vi "Delete.vi"(8 "error in":errorcluster caption="错误输入（无错误）", 10 "Data":variant, 11 "PanelRootNode 输入":refnum<class "PanelRootNode.lvclass"> caption="DNL_LabVIEW Object in") -> (0 "error out":errorcluster caption="错误输出", 3 "PanelRootNode 输出":refnum<class "PanelRootNode.lvclass"> caption="DNL_LabVIEW Object out")   [LabVIEW 2013, in "PanelRootNode.lvclass"]
uses:
  PanelRootNode.lvclass
  PanelObject/PanelObject.lvclass
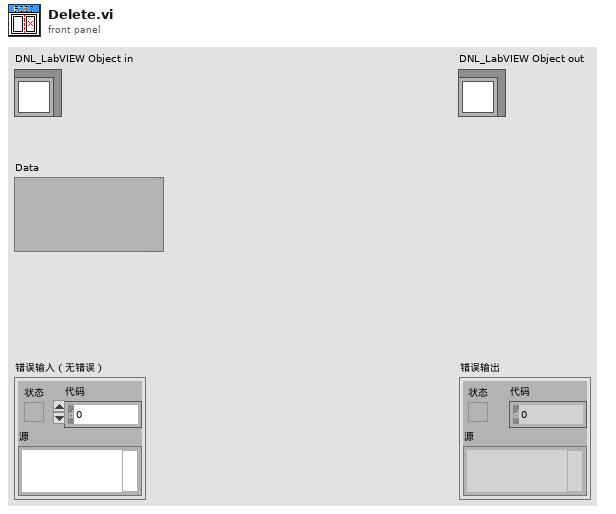
[diagram p1: front panel]
types:
  T1 = cluster{"Node*":refnum<data-value>, "AbortVI":bool}
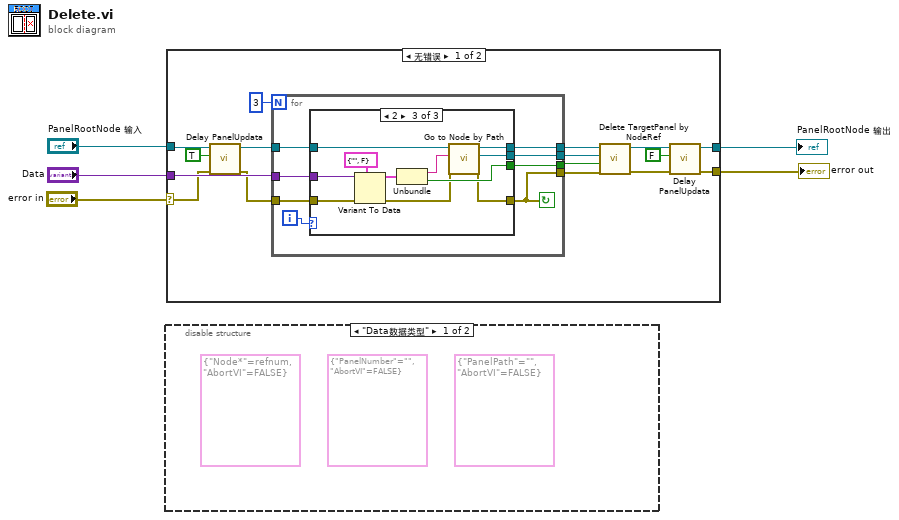
[diagram p0: block diagram]
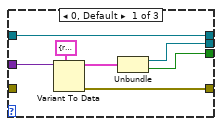
[diagram p3: hidden frame]
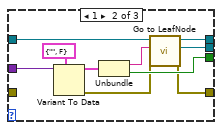
[diagram p4: hidden frame]
diagram:
  n1 = disable-structure shown="\"Data数据类型\"" {
    frame condition #0 {
      (unwired) cluster{"PanelPath":string, "AbortVI":bool} {"PanelPath"="", "AbortVI"=FALSE}
      (unwired) cluster{"PanelNumber":string, "AbortVI":bool} {"PanelNumber"="", "AbortVI"=FALSE}
      (unwired) T1 {"Node*"=refnum, "AbortVI"=FALSE}
    }
    frame condition #1 (active) {
    }
  }
  n2 = case shown="无错误" "error in" {
    selector: "error in" -> [w13 w59]
    tunnel: [w8 w59] -> w4
    tunnel: [w7 w58] -> w2
    tunnel: "PanelRootNode 输入" -> [w15 w58]
    tunnel: "Data" -> [w20 _]
    frame No Error {
      n3 = call "Delay PanelUpdata.vi"("error in (no error)"=w13, "延迟前面板更新"=TRUE, "PanelRootNode 输入"=w15) -> ("error out"=w12:errorcluster, "PanelRootNode 输出"=w14:refnum<class "PanelRootNode.lvclass">)  [unwired: 7 in]
      n4 = for {
        N: 3 -> [_]
        tunnel: [w28] -> w19
        tunnel: [w27] -> w17
        tunnel: w14 -> [w26]
        tunnel: [w25] -> w16
        tunnel: [w24] -> w18
        tunnel: w20 -> [w23]
        tunnel: w12 -> [w22]
        i -> [w29]
        stop <- w24 continue-if-true
        n5 = case shown="2" w29 {
          tunnel: [w36 w46 w57] -> w25
          tunnel: [w35 w42 w53] -> w27
          tunnel: [w32 w44 w55] -> w28
          tunnel: [w33 w41 w52] -> w24
          tunnel: w26 -> [w32 w39 w51]
          tunnel: w23 -> [w31 w38 w49]
          tunnel: w22 -> [_ _ w47]
          frame 0, Default {
            n6 = Variant To Data(type=T1 {"Node*"=refnum, "AbortVI"=FALSE}, Variant=w31) -> (data=w34:T1, error out=w33:errorcluster)  [unwired: 1 in]
            n7 = Unbundle(w34) -> ("Node*"=w35:refnum<data-value>, "AbortVI"=w36:bool)
          }
          frame 1 {
            n8 = Variant To Data(type=cluster{"PanelNumber":string, "AbortVI":bool} {"PanelNumber"="", "AbortVI"=FALSE}, Variant=w38) -> (data=w45:cluster{"PanelNumber":string, "AbortVI":bool}, error out=w40:errorcluster)  [unwired: 1 in]
            n9 = Unbundle(w45) -> ("PanelNumber"=w43:string, "AbortVI"=w46:bool)
            n10 = call-dynamic "Go to LeafNode.vi"("error in"=w40, "LeafNumber"=w43, "PanelRootNode 输入"=w39) -> ("error out"=w41:errorcluster, "Node*"=w42:refnum<data-value>, "PanelRootNode 输出"=w44:refnum<class "PanelRootNode.lvclass">)  [unwired: 5 in, 1 out]
          }
          frame 2 {
            n11 = Variant To Data(error in=w47, type=cluster{"PanelPath":string, "AbortVI":bool} {"PanelPath"="", "AbortVI"=FALSE}, Variant=w49) -> (data=w56:cluster{"PanelPath":string, "AbortVI":bool}, error out=w50:errorcluster)
            n12 = Unbundle(w56) -> ("PanelPath"=w54:string, "AbortVI"=w57:bool)
            n13 = call-dynamic "Go to Node by Path.vi"("error in"=w50, "NodePath"=w54, "PanelLinkNode 输入"=w51) -> ("error out"=w52:errorcluster, "Node*"=w53:refnum<data-value>, "PanelLinkNode 输出"=w55:refnum<class "PanelRootNode.lvclass">)  [unwired: 5 in, 1 out]
          }
        }
      }
      n14 = call-dynamic "Delete TargetPanel by NodeRef.vi"("error in"=w18, "Abort VI"=w16, "Node*"=w17, "PanelRootNode 输入"=w19) -> ("error out"=w10:errorcluster, "PanelRootNode 输出"=w9:refnum<class "PanelRootNode.lvclass">)  [unwired: 6 in]
      n15 = call "Delay PanelUpdata.vi"("error in (no error)"=w10, "延迟前面板更新"=FALSE, "PanelRootNode 输入"=w9) -> ("error out"=w8:errorcluster, "PanelRootNode 输出"=w7:refnum<class "PanelRootNode.lvclass">)  [unwired: 7 in]
    }
    frame Error {
    }
  }
  "error out" <- w4
  "PanelRootNode 输出" <- w2
